vi "Escape Chars Defs.vi"() -> (3 "Escapes":cluster{"String":string, "Escape":string}[](array[cluster]))   [LabVIEW 2020, in "NI_VIAnCFGDataStructure.lvlib" / "Tree.lvclass"]
doc: "This is the definition of the characters used to escape the strings for String Tree Data types. Use this list for information purposes. Modifying the list in this VI will make the String Tree Data types function differently."
uses:
  <vilib>/addons/analyzer/VIAnCFGDataStructure/Tree Manager/Tree.lvclass
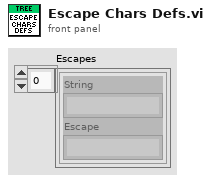
[diagram p1: front panel]
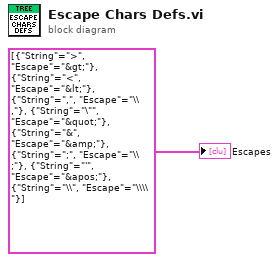
[diagram p0: block diagram]
diagram:
  "Escapes" <- cluster{"String":string, "Escape":string}[] [{"String"=">", "Escape"="&gt;"}, {"String"="<", "Escape"="&lt;"}, {"String"=",", "Escape"="\\,"}, {"String"="\"", "Escape"="&quot;"}, {"String"="&", "Escape"="&amp;"}, {"String"=";", "Escape"="\\;"}, {"String"="'", "Escape"="&apos;"}, {"String"="\\", "Escape"="\\\\"}] ("Escapes")
